vi "LVH5TMajorErrorEquals.vi"(8 "error in":errorcluster, 10 "error num":i32, 11 "major_id":T1) -> (0 "error out":errorcluster, 3 "equals?":bool)   [LabVIEW 2017]
uses:
  <vilib>/UPVI/lvhdf5/error.llb/LVH5EMajorID.ctl
panel:
  # "LVHDF5 Toolkit\nCopyright (c) 2005-2013 by Jason D. Sommerville\nCopyright (c) 2014 by UPVI, LLC.\n\nThis use and distribution of this file is governed by the terms found in \nLICENSE.txt distributed with this toolkit and installed at\n <user.lib>\\_lvhdf5\\LICENSE.txt"
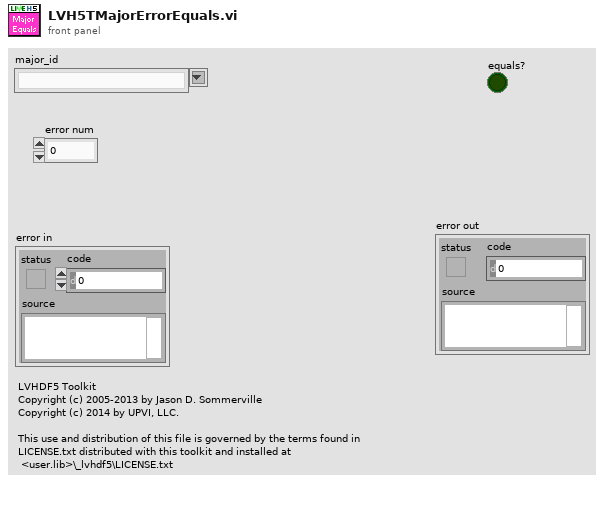
[diagram p1: front panel]
types:
  T1 = typedef "LVH5EMajorID.ctl" = string
  T2 = typedef "HDF5 Ref.ctl" = refnum<k1>
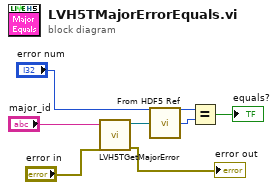
[diagram p0: block diagram]
diagram:
  n1 = call <vilib>:"LVH5TGetMajorError.vi"("error in"="error in", "major_id"="major_id") -> ("error out"=→"error out":errorcluster, "HDF5 Ref"=w5:T2)  [unwired: 8 in]
  n2 = call <vilib>:"From HDF5 Ref.vi"("HDF5 Ref"=w5) -> ("I32"=w4:i32)
  n3 = Equal?(x="error num", y=w4) -> (x = y?=→"equals?":bool)
